vi "VCS Set Controller Gain.vi"(8 "error in (no error)":errorcluster, 9 "value":u64, 10 "controller gain":cluster{"controller":u16, "gain":u16}={"controller"=1, "gain"=1} {"gain" items=["P-Gain"=1, "I-Gain"=2, "D-Gain"=3, "Feedforward Velocity Gain"=10, "Feedforward Acceleration Gain"=11, "Theta Gain"=20, "Omega Gain"=21, "Tau Gain"=22, "P Gain low"=101, "P Gain high"=102, "Gain Scheduling Weight"=110, "Filter Coefficient A"=120, "Filter Coefficient B"=121, "Filter Coefficient C"=122, "Filter Coefficient D"=123, "Filter Coefficient E"=124]; "controller" items=["PI Current Controller"=1, "PI Velocity Controller"=10, "PI Velocity Controller with Observer"=11, "PID Position Controller"=20, "Dual Loop Position Controller"=21]}, 11 "axis in":cluster{"keyHandle":u32, "nodeId":u16}={"keyHandle"=0, "nodeId"=1}) -> (0 "error out":errorcluster, 3 "axis out":cluster{"keyHandle":u32, "nodeId":u16}={"keyHandle"=0, "nodeId"=1})   [LabVIEW 2019, in "maxonEPOS.lvlib"]
doc: "<B>VCS Get Current Regulator Gain</B> reads all current regulator gains."
uses:
  Examples/maxonEPOS.lvlib
  Resources/EposCmd64.dll
  Resources/EposCmd.dll
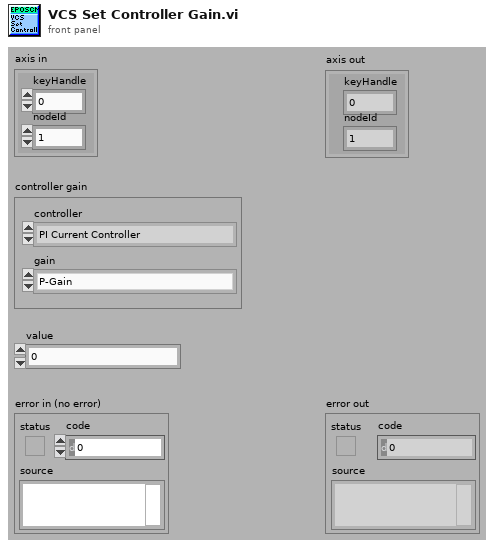
[diagram p1: front panel]
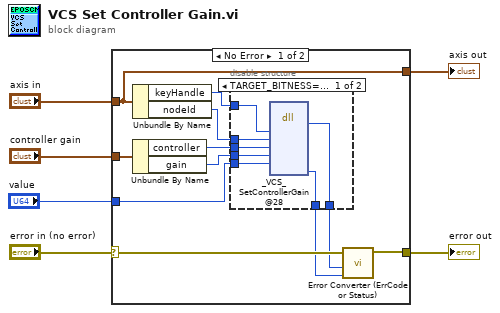
[diagram p0: block diagram]
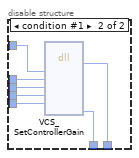
[diagram p2: hidden frame]
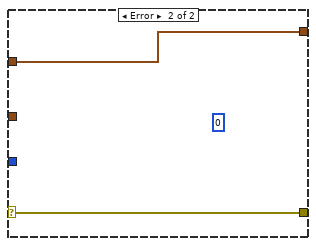
[diagram p3: hidden frame]
diagram:
  n1 = case shown="No Error" "error in (no error)" {
    selector: "error in (no error)" -> [w17 w33]
    tunnel: [w16 w33] -> w5
    tunnel: "axis in" -> [w12 w32]
    tunnel: [w12 w32] -> w3
    tunnel: "controller gain" -> [w10 _]
    tunnel: "value" -> [w7 _]
    frame No Error {
      n2 = Unbundle By Name(w12) -> ("keyHandle"=w14:u32, "nodeId"=w13:u16)
      n3 = Unbundle By Name(w10) -> ("controller"=w9:u16, "gain"=w8:u16)
      n4 = disable-structure shown="TARGET_BITNESS==32, Standard" {
        disable-tunnel: [w24 w31] -> w15
        disable-tunnel: w14 -> [w23 w30]
        disable-tunnel: w13 -> [w22 w29]
        disable-tunnel: [w21 w28] -> w11
        disable-tunnel: w7 -> [w20 w27]
        disable-tunnel: w9 -> [w19 w26]
        disable-tunnel: w8 -> [w18 w25]
        frame condition #0 (active) {
          n5 = dll-call lib="C:/workspace/project/scancon/sw/SSI_Tool/InstrumentsInterfaces/Motordriver/maxon EPOS/Resources/EposCmd.*" fn="_VCS_SetControllerGain@28" ("EposCmd.dll:_VCS_GetCurrentRegulatorGain@20")("KeyHandle"=w23, "NodeId"=w22, "Controller"=w19, "Gain"=w18, "Value"=w20) -> ("Rückgabetyp"=w21:i32, "pErrorCode"=w24:u32)  [unwired: 9 in, 2 out]
        }
        frame condition #1 {
          n6 = dll-call lib="C:/Sources/LabView/maxon EPOS/Resources/EposCmd64.dll" fn="VCS_SetControllerGain" ("EposCmd.dll:_VCS_GetCurrentRegulatorGain@20")("KeyHandle"=w30, "NodeId"=w29, "Controller"=w26, "Gain"=w25, "Value"=w27) -> ("Rückgabetyp"=w28:i32, "pErrorCode"=w31:u32)  [unwired: 9 in, 2 out]
        }
      }
      n7 = call "Error Converter (ErrCode or Status).vi"("error code"=w15, "return type"=w11, "error in (no error)"=w17) -> ("error out"=w16:errorcluster)  [unwired: 7 in]
    }
    frame Error {
      (unwired) u64 0 ("pI")
    }
  }
  "error out" <- w5
  "axis out" <- w3
